vi "Project Manager Is Process Running.vi"(7 "Exe Number":i32, 8 "Error In":errorcluster, 9 "Station Group":T1, 10 "Newfi Search":string="Newfi", 11 "2015 Search":string="2015_") -> (0 "Error Out":errorcluster, 1 "Viper/Hawk Unit":bool, 2 "2015 Unit":bool, 3 "Process is Already Running":bool, 4 "2015 Array":string[](array[string]), 5 "2015 Search String":string, 6 "Newfi Array":string[](array[string]))   [LabVIEW 2014]
uses:
  Washer HCC/Washer HCC NEWFI/Type Definitions/HCC Station Group.ctl
panel:
  out "Viper/Hawk Search String":string
  out "procese":string[](array[string])
  # "Determine if the process\nis already running"
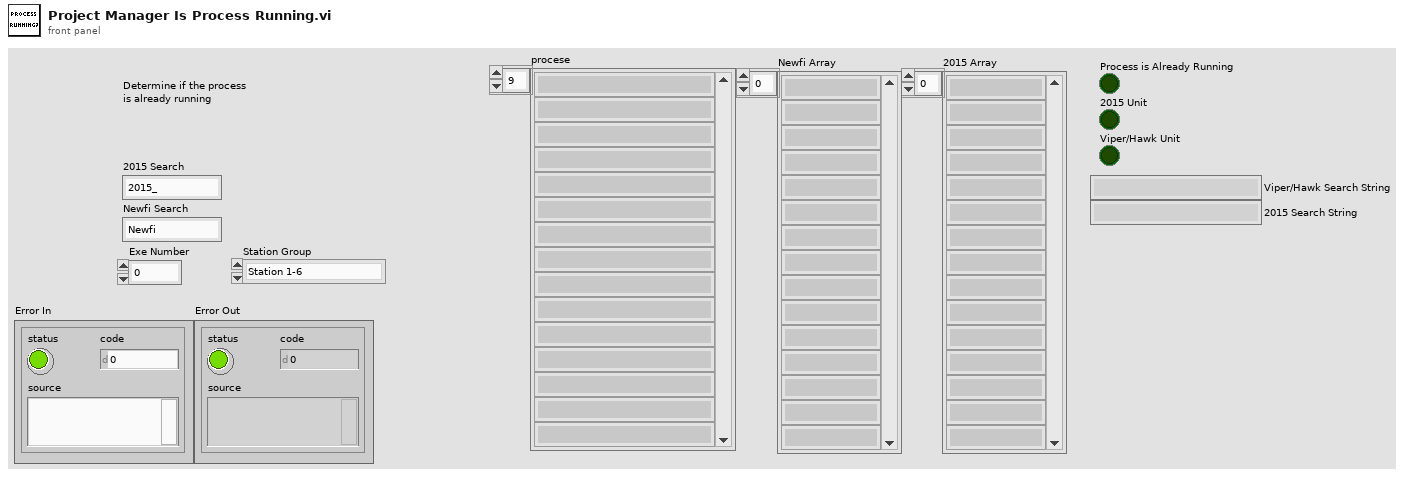
[diagram p1: front panel]
types:
  T1 = typedef "HCC Station Group.ctl" = enum16{"Station 1-6", "Station 7-12", "Station 13-18", "Station 19-24"}
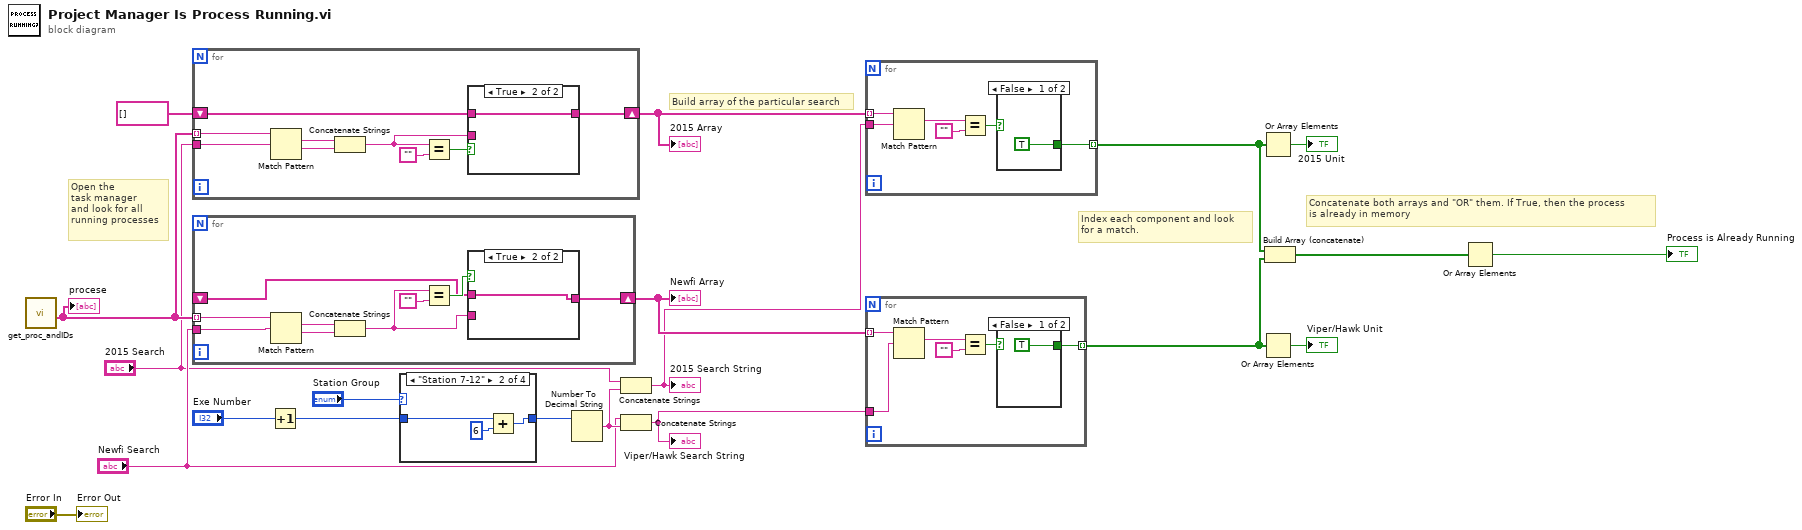
[diagram p0: block diagram]
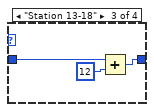
[diagram p3: hidden frame]
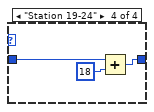
[diagram p4: hidden frame]
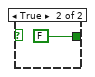
[diagram p5: hidden frame]
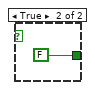
[diagram p6: hidden frame]
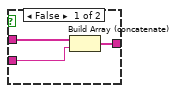
[diagram p7: hidden frame]
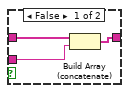
[diagram p8: hidden frame]
diagram:
  # "Build array of the particular search"
  # "Concatenate both arrays and \"OR\" them. If True, then the process\nis already in memory"
  # "Index each component and look\nfor a match."
  # "Open the \ntask manager\nand look for all \nrunning processes"
  n1 = call "get_proc_andIDs.vi"() -> ("procese"=w18:string[])  [unwired: 11 out]
  "procese" <- w18
  n2 = for {
    tunnel: w18 -> [w29] mode=indexing
    shift-right: [w23] -> w17
    shift-left: string[] [] -> [w24]
    tunnel: "2015 Search" -> [w21]
    n3 = Match Pattern(string=w29, regular expression=w21) -> (match substring=w28:string, after substring=w27:string)  [unwired: 1 in, 2 out]
    n4 = Concatenate Strings(w28, w27) -> (w22:string)
    n5 = Equal?(x=w22, y="") -> (x = y?=w26:bool)
    n6 = case shown="True" w26 {
      tunnel: w24 -> [w32 w33]
      tunnel: [w31 w33] -> w23
      tunnel: w22 -> [w30 _]
      frame False {
        n7 = Build Array (concatenate)(w32, w30) -> (w31:string[])
      }
      frame True {
      }
    }
  }
  "2015 Array" <- w17
  n8 = for {
    tunnel: w18 -> [w42] mode=indexing
    shift-right: [w36] -> w15
    shift-left: _ -> [w37]
    tunnel: "Newfi Search" -> [w34]
    n9 = Match Pattern(string=w42, regular expression=w34) -> (match substring=w41:string, after substring=w40:string)  [unwired: 1 in, 2 out]
    n10 = Concatenate Strings(w41, w40) -> (w35:string)
    n11 = Equal?(x=w35, y="") -> (x = y?=w39:bool)
    n12 = case shown="True" w39 {
      tunnel: w37 -> [w45 w46]
      tunnel: [w44 w46] -> w36
      tunnel: w35 -> [w43 _]
      frame False {
        n13 = Build Array (concatenate)(w45, w43) -> (w44:string[])
      }
      frame True {
      }
    }
  }
  "Newfi Array" <- w15
  n14 = Increment(x="Exe Number") -> (x+1=w2:i32)
  n15 = case shown="\"Station 7-12\"" "Station Group" {
    tunnel: w2 -> [w47 w49 w52 w55]
    tunnel: [w47 w48 w51 w54] -> w1
    frame "Station 1-6", Default {
    }
    frame "Station 7-12" {
      n16 = Add(x=w49, y=6 ("size(s)")) -> (x+y=w48:i32)
    }
    frame "Station 13-18" {
      n17 = Add(x=w52, y=12 ("size(s)")) -> (x+y=w51:i32)
    }
    frame "Station 19-24" {
      n18 = Add(x=w55, y=18 ("size(s)")) -> (x+y=w54:i32)
    }
  }
  n19 = Number To Decimal String(number=w1) -> (decimal integer string=w16:string)  [unwired: 1 in]
  n20 = Concatenate Strings("2015 Search", w16) -> (w13:string)
  "2015 Search String" <- w13
  n21 = Concatenate Strings("Newfi Search", w16) -> (w14:string)
  "Viper/Hawk Search String" <- w14
  n22 = for {
    tunnel: w17 -> [w62] mode=indexing
    tunnel: w13 -> [w61]
    tunnel: [w57] -> w10 mode=indexing
    n23 = Match Pattern(string=w62, regular expression=w61) -> (match substring=w59:string)  [unwired: 1 in, 3 out]
    n24 = Equal?(x=w59, y="") -> (x = y?=w60:bool)
    n25 = case shown="False" w60 {
      tunnel: [TRUE FALSE] -> w57
      frame False {
      }
      frame True {
      }
    }
  }
  n26 = for {
    tunnel: w15 -> [w70] mode=indexing
    tunnel: w14 -> [w69]
    tunnel: [w65] -> w9 mode=indexing
    n27 = Match Pattern(string=w70, regular expression=w69) -> (match substring=w67:string)  [unwired: 1 in, 3 out]
    n28 = Equal?(x=w67, y="") -> (x = y?=w66:bool)
    n29 = case shown="False" w66 {
      tunnel: [TRUE FALSE] -> w65
      frame False {
      }
      frame True {
      }
    }
  }
  n30 = Or Array Elements(Boolean array=w10) -> (logical OR=→"2015 Unit":bool)
  n31 = Or Array Elements(Boolean array=w9) -> (logical OR=→"Viper/Hawk Unit":bool)
  n32 = Build Array (concatenate)(w10, w9) -> (w12:bool[])
  n33 = Or Array Elements(Boolean array=w12) -> (logical OR=→"Process is Already Running":bool)
  "Error Out" <- "Error In"
